vi "Heater Construct.vi"() -> ()   [LabVIEW 2015]
panel:
  in  "PID 2":cluster{"P":dbl, "I":dbl, "D":dbl}={"P"=200.0, "I"=4.0, "D"=100.0}
  in  "Setpoint 2":dbl=30.0 format="%#_13g"
  out "Waveform Chart 2":i16(graph)
  in  "ON 2":bool
  in  "ON":bool
  out "Waveform Chart":i16(graph)
  in  "Setpoint":dbl=30.0 format="%#_13g"
  in  "PID":cluster{"P":dbl, "I":dbl, "D":dbl}={"P"=200.0, "I"=4.0, "D"=100.0}
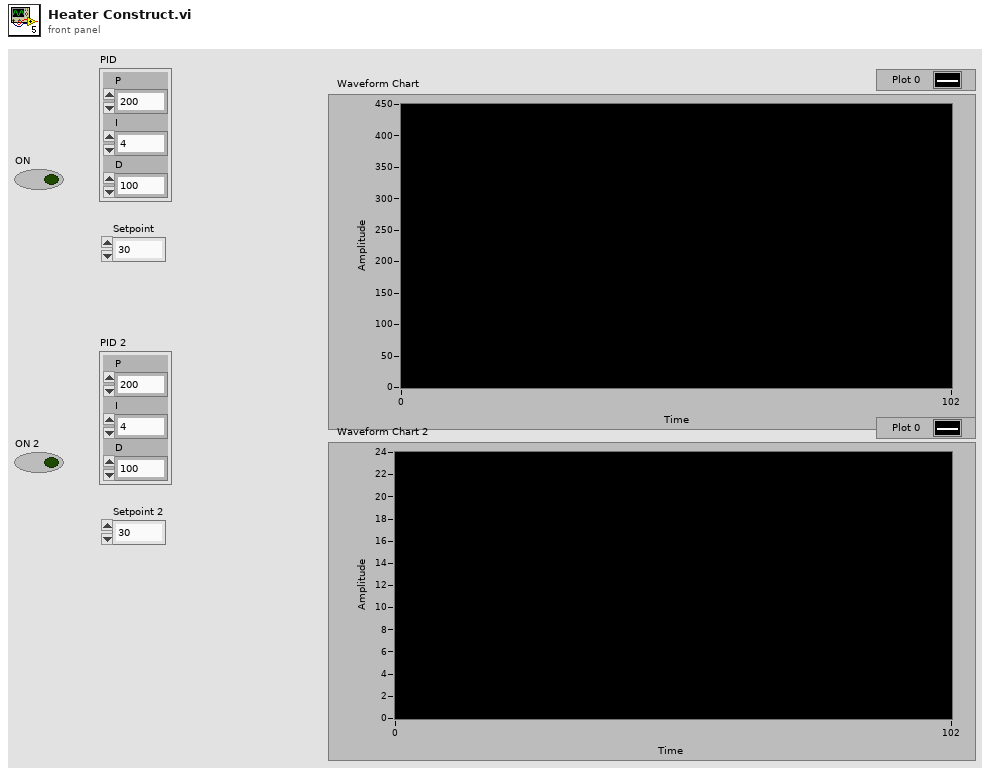
[diagram p1: front panel]
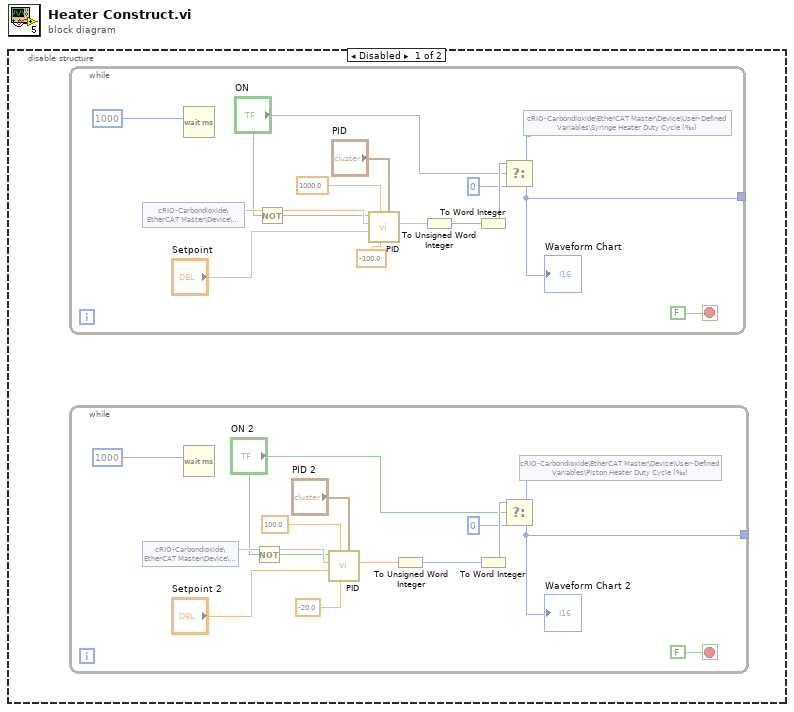
[diagram p0: block diagram]
diagram:
  n1 = disable-structure shown="Disabled" {
    frame Disabled {
      n2 = while {
        tunnel: [w15] -> _
        stop <- FALSE stop-if-true
        n3 = shared-variable "cRIO-Carbondioxide\\EtherCAT Master\\Device\\Mod2\\Syringe TC"() -> (w23:dbl)  [unwired: 1 in, 1 out]
        n4 = Wait (ms)(milliseconds to wait=u32 1000) -> ()  [unwired: 1 out]
        n5 = Not(x="ON") -> (.not. x?=w18:bool)
        n6 = call "PID.vi"("PID"="PID", "Lower Limit"=-100.0, "Upper Limit (0,01)"=1000.0, "Setpoint (0,002)"="Setpoint", "Process"=w23, "Reset"=w18) -> ("Output"=w20:dbl)  [unwired: 4 in, 1 out]
        n7 = To Unsigned Word Integer(number=w20) -> (unsigned 16bit integer=w17:u16)
        n8 = To Word Integer(number=w17) -> (16bit integer=w22:i16)
        n9 = Select(t=w22, s="ON", f=i16 0 ("t")) -> (s? t:f=w15:i16)
        "Waveform Chart" <- w15
        n10 = shared-variable "cRIO-Carbondioxide\\EtherCAT Master\\Device\\User-Defined Variables\\Syringe Heater Duty Cycle (‰)"(w15) -> ()  [unwired: 1 in, 1 out]
      }
      n11 = while {
        tunnel: [w1] -> _
        stop <- FALSE stop-if-true
        n12 = shared-variable "cRIO-Carbondioxide\\EtherCAT Master\\Device\\Mod2\\Piston TC"() -> (w8:dbl)  [unwired: 1 in, 1 out]
        n13 = Wait (ms)(milliseconds to wait=u32 1000) -> ()  [unwired: 1 out]
        n14 = Not(x="ON 2") -> (.not. x?=w4:bool)
        n15 = call "PID.vi"("PID"="PID 2", "Lower Limit"=-20.0, "Upper Limit (0,01)"=100.0, "Setpoint (0,002)"="Setpoint 2", "Process"=w8, "Reset"=w4) -> ("Output"=w3:dbl)  [unwired: 4 in, 1 out]
        n16 = To Unsigned Word Integer(number=w3) -> (unsigned 16bit integer=w2:u16)
        n17 = To Word Integer(number=w2) -> (16bit integer=w7:i16)
        n18 = Select(t=w7, s="ON 2", f=i16 0 ("t")) -> (s? t:f=w1:i16)
        "Waveform Chart 2" <- w1
        n19 = shared-variable "cRIO-Carbondioxide\\EtherCAT Master\\Device\\User-Defined Variables\\Piston Heater Duty Cycle (‰)"(w1) -> ()  [unwired: 1 in, 1 out]
      }
    }
    frame Enabled {
    }
  }
